vi "BuildFullTag.vi"(7 "Menu Ref":refnum<data-value>, 8 "error in (no error)":errorcluster, 9 "Build Full Tree":bool, 10 "Parent Tag":string, 11 "MGI_MenuItem in":refnum<class "MGI_MenuItem.lvclass">) -> (0 "error out":errorcluster, 3 "MGI_MenuItem out":refnum<class "MGI_MenuItem.lvclass">)   [LabVIEW 2016, in "MGI_MenuItem.lvclass"]
doc: "Builds the full tag. A full tag gives a full path from the parent to the children. It is used when identifying which menu item has been clicked.\n\nAuthored by Derek E. Trepanier\nsupport@mooregoodideas.com\nwww.mooregoodideas.com\n\nCopyright (c) 2012, Moore Good Ideas, Inc.\n\nAll rights reserved.\n\nRedistribution and use in source and binary forms, with or without modification, are permitted provided that the following conditions are met:\n\n * Redistributions of source code must retain the above copyright notice, this list of conditions and the following disclaimer.\n * Redistributions in binary form must reproduce the above copyright notice, this list of conditions and the following disclaimer in the documentation and/or other materials provided with the distribution.\n * Neither the name of Moore Good Ideas, Inc. nor the names of its contributors may be used to endorse or promote products derived from this software without specific prior written permission.\n\nTHIS SOFTWARE IS PROVIDED BY THE COPYRIGHT HOLDERS AND CONTRIBUTORS \"AS IS\" AND ANY EXPRESS OR IMPLIED WARRANTIES, INCLUDING, BUT NOT LIMITED TO, THE IMPLIED WARRANTIES OF MERCHANTABILITY AND FITNESS FOR A PARTICULAR PURPOSE ARE DISCLAIMED. IN NO EVENT SHALL THE COPYRIGHT OWNER OR CONTRIBUTORS BE LIABLE FOR ANY DIRECT, INDIRECT, INCIDENTAL, SPECIAL, EXEMPLARY, OR CONSEQUENTIAL DAMAGES (INCLUDING, BUT NOT LIMITED TO, PROCUREMENT OF SUBSTITUTE GOODS OR SERVICES; LOSS OF USE, DATA, OR PROFITS; OR BUSINESS INTERRUPTION) HOWEVER CAUSED AND ON ANY THEORY OF LIABILITY, WHETHER IN CONTRACT, STRICT LIABILITY, OR TORT (INCLUDING NEGLIGENCE OR OTHERWISE) ARISING IN ANY WAY OUT OF THE USE OF THIS SOFTWARE, EVEN IF ADVISED OF THE POSSIBILITY OF SUCH DAMAGE."
uses:
  <userlib>/_MGI/Menu Building/MenuItem/MGI_MenuItem.lvclass
  <userlib>/_MGI/Menu Building/MenuTypes/MGI_Menu.lvclass
  <userlib>/_MGI/Menu Building/MenuItem/MGI_MenuItem.lvclass/MGI_MenuItem.ctl
  <userlib>/_MGI/Menu Building/MenuItem/Read Sub-Menus.vi
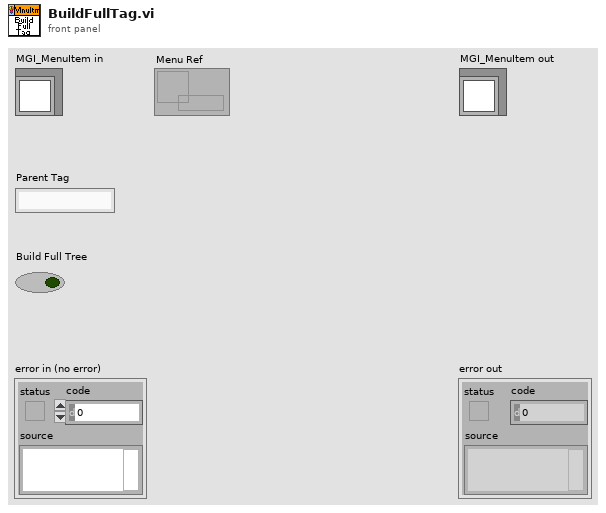
[diagram p1: front panel]
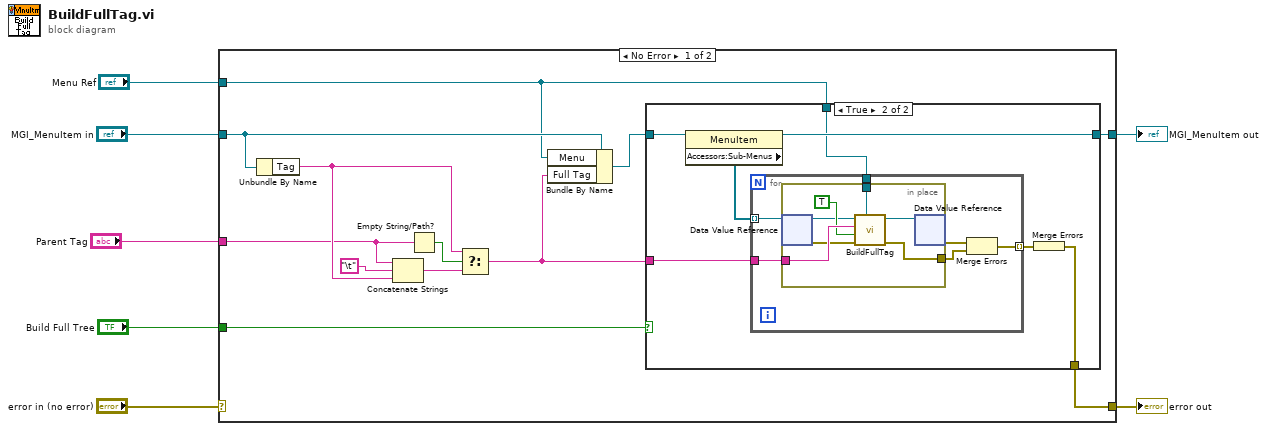
[diagram p0: block diagram]
diagram:
  n1 = case shown="No Error" "error in (no error)" {
    selector: "error in (no error)" -> [_ w42]
    tunnel: [w10 w42] -> w6
    tunnel: [w14 w41] -> w4
    tunnel: "MGI_MenuItem in" -> [w17 w41]
    tunnel: "Parent Tag" -> [w15 _]
    tunnel: "Build Full Tree" -> [w12 _]
    tunnel: "Menu Ref" -> [w8 _]
    frame No Error {
      n2 = Unbundle By Name(w17) -> ("Tag"=w16:string)
      n3 = Concatenate Strings(w15, "\t", w16) -> (w19:string)
      n4 = Empty String/Path?(string/path=w15) -> (empty?=w18:bool)
      n5 = Select(t=w16, s=w18, f=w19) -> (s? t:f=w11:string)
      n6 = Bundle By Name(cluster=w17, "Menu"=w8, "Full Tag"=w11) -> (w13:refnum<class "MGI_MenuItem.lvclass">)
      n7 = case shown="True" w12 {
        tunnel: [w20 w25] -> w14
        tunnel: w13 -> [w20 w26]
        tunnel: w11 -> [_ w27]
        tunnel: [_ w22] -> w10
        tunnel: w8 -> [_ w21]
        frame False {
        }
        frame True {
          n8 = property class="MenuItem"(reference=w26) -> (reference out=w25:refnum<class "MGI_MenuItem.lvclass">, "Accessors:Sub-Menus"=w24:refnum<data-value>[])  [unwired: 1 in, 1 out]
          n9 = for {
            tunnel: w27 -> [w33]
            tunnel: w24 -> [w31] mode=indexing
            tunnel: [w30] -> w23 mode=indexing
            tunnel: w21 -> [w28]
            n10 = in-place {
              in-place-border: w33 -> [w40]
              in-place-border: [w38] -> w32
              in-place-border: w28 -> [w34]
              n11 = in-place-dvr #1(w31) -> (w37:refnum<class "MGI_MenuItem.lvclass">, w35:errorcluster)
              n12 = call <userlib>:"BuildFullTag.vi"("Menu Ref"=w34, "error in (no error)"=w35, "Build Full Tree"=TRUE, "Parent Tag"=w40, "MGI_MenuItem in"=w37) -> ("error out"=w38:errorcluster, "MGI_MenuItem out"=w36:refnum<class "MGI_MenuItem.lvclass">)  [unwired: 5 in]
              n13 = in-place-dvr #1(w36) -> (w29:errorcluster)  [unwired: 1 out]
            }
            n14 = Merge Errors(w29, w32) -> (w30:errorcluster)
          }
          n15 = Merge Errors(w23) -> (w22:errorcluster)
        }
      }
    }
    frame Error {
    }
  }
  "error out" <- w6
  "MGI_MenuItem out" <- w4
